vi "Calcuate Stage PSD.vi"() -> ()   [LabVIEW 2014]
uses:
  <vilib>/Utility/file.llb/Read From Spreadsheet File (DBL).vi
panel:
  in  "Filter type":T1(ring)
  in  "Avg points":i32
  in  "Tab Control":enum32{"Page 1", "Page 2"}(tab)
  out "Waveform Graph":dbl[][](graph)
  out "XY Graph":T2(graph)
  in  "T=NI made PSD\nF=YCC made PSD":bool
  in  "Time per avg":dbl
  in  "Data rate (Hz)":dbl
  out "first row":dbl[](array[numeric]) format="%0.3f"
  in  "file path (dialog if empty)":path
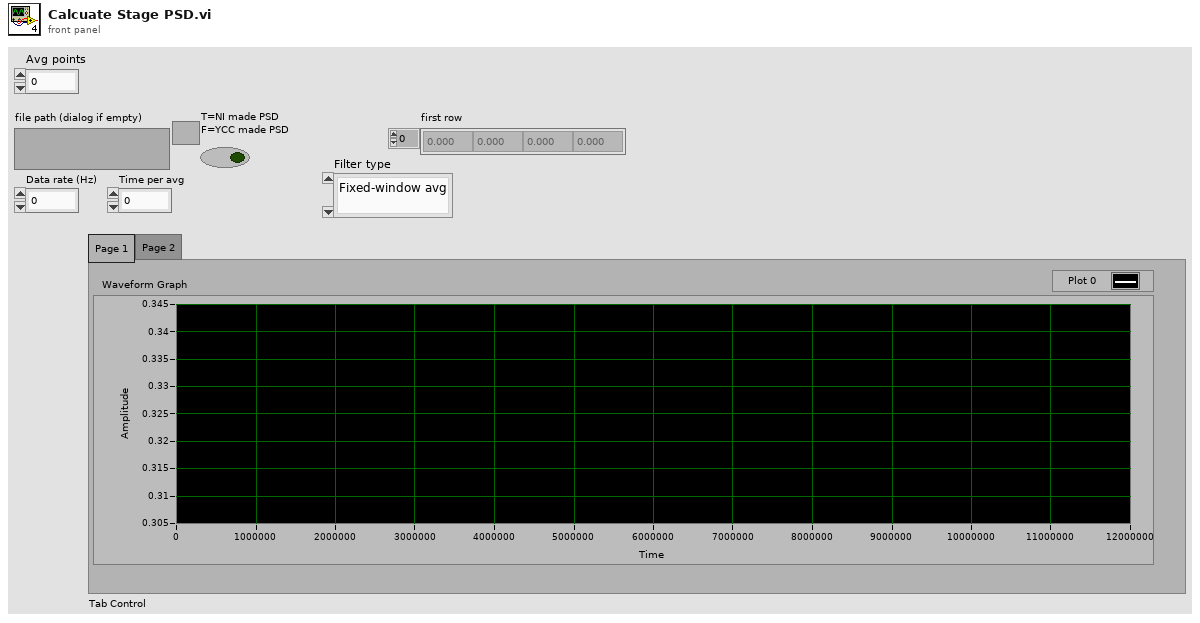
[diagram p1: front panel]
types:
  T1 = enum16{"Fixed-window avg", "Moving-window avg", "F+S-window avg", "S-G filter", "Fixed-window Median", "Moving-window Median "}
  T2 = cluster{"Frequency (Hz)\n0,df, 2df,...(n/2-1)Fs":dbl[], "Avg. PSD":dbl[]}
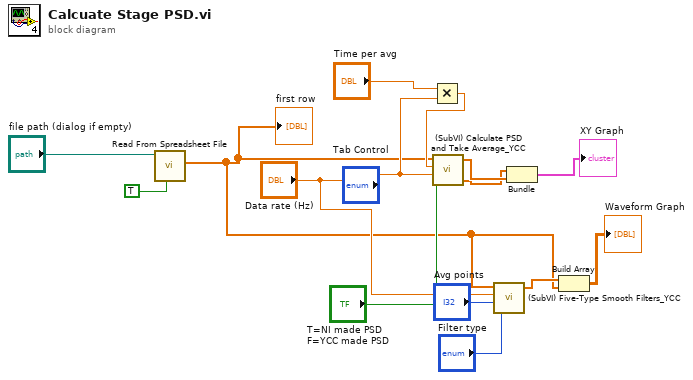
[diagram p0: block diagram]
diagram:
  n1 = call-poly <vilib>:"Read From Spreadsheet File.vi"("transpose (no:F)"=TRUE, "file path (dialog if empty)"="file path (dialog if empty)") -> ("first row"=w3:dbl[])  [unwired: 5 in, 4 out]
  "first row" <- w3
  n2 = Multiply(x="Time per avg", y="Data rate (Hz)") -> (x*y=w12:dbl)
  n3 = call "(SubVI) Calculate PSD and Take Average_YCC.vi"("Data"=w3, "#samples per avg"=w12, "Data rate (Hz)"="Data rate (Hz)", "T=NI made PSD\nF=YCC made PSD"="T=NI made PSD\nF=YCC made PSD") -> ("Avg. PSD"=w10:dbl[], "Frequency (Hz)\n0,df, 2df,...(n/2-1)Fs"=w9:dbl[])  [unwired: 3 in]
  n4 = call "(SubVI) Five-Type Smooth Filters_YCC.vi"("Filter type"="Filter type", "Avg points"="Avg points", "Sampling rate (Hz)"="Data rate (Hz)", "QPD data"=w3) -> ("Filtered QPD data"=w4:dbl[])  [unwired: 1 in, 1 out]
  n5 = Bundle("Frequency (Hz)\n0,df, 2df,...(n/2-1)Fs"=w9, "Avg. PSD"=w10) -> (→"XY Graph":T2)  [unwired: 1 in]
  n6 = Build Array(w4, w3) -> (→"Waveform Graph":dbl[][])
